vi "get_max_min.vi"(8 "error in":errorcluster, 11 "PI P123.01 & PiezoDrive TD250 & NI USB 7855R.lvclass":refnum<class "PI P123.01 & PiezoDrive TD250 & NI USB 7855R.lvclass">) -> (0 "error out":errorcluster, 1 "Piezo_minimum":i16, 2 "Piezo_maximum":i16, 3 "PI P123.01 & PiezoDrive TD250 & NI USB 7855R.lvclass 2":refnum<class "PI P123.01 & PiezoDrive TD250 & NI USB 7855R.lvclass">)   [LabVIEW 2020, in "PI P123.01 & PiezoDrive TD250 & NI USB 7855R.lvclass"]
uses:
  PI P123.01 & PiezoDrive TD250 & NI USB 7855R.lvclass
  PI P123.01 & PiezoDrive TD250 & NI USB 7855R.lvclass/PI P123.01 & PiezoDrive TD250 & NI USB 7855R.ctl
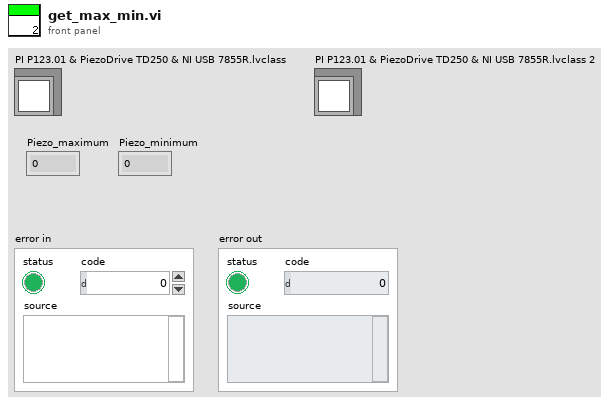
[diagram p1: front panel]
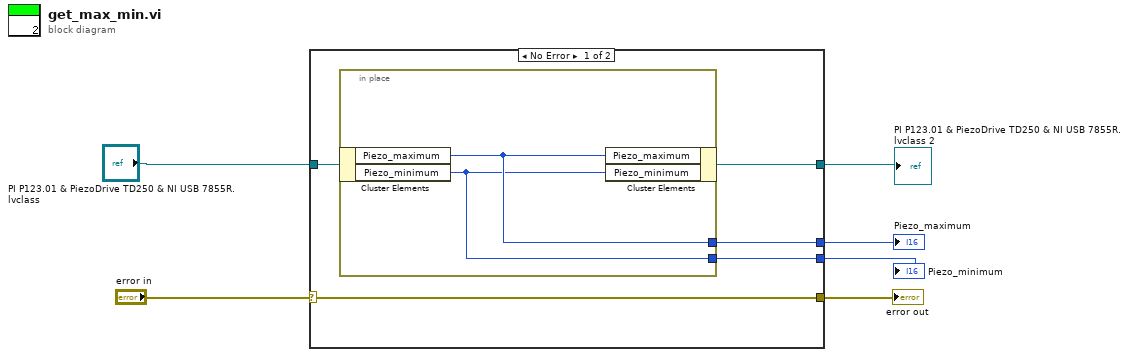
[diagram p0: block diagram]
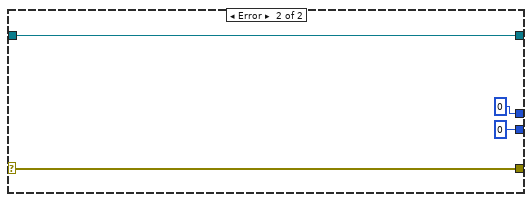
[diagram p2: hidden frame]
diagram:
  n1 = case shown="No Error" "error in" {
    selector: "error in" -> [w9 w16]
    tunnel: "PI P123.01 & PiezoDrive TD250 & NI USB 7855R.lvclass" -> [w11 w17]
    tunnel: [w10 w17] -> w5
    tunnel: [w9 w16] -> w3
    tunnel: [w8 i16 0 ("Piezo_maximum")] -> w2
    tunnel: [w7 i16 0 ("Piezo_minimum")] -> w1
    frame No Error {
      n2 = in-place {
        in-place-border: [w13] -> w8
        in-place-border: [w12] -> w7
        n3 = in-place-cluster #1(w11) -> ("Piezo_maximum"=w13:i16, "Piezo_minimum"=w12:i16)
        n4 = in-place-cluster #1("Piezo_maximum"=w13, "Piezo_minimum"=w12) -> (w10:refnum<class "PI P123.01 & PiezoDrive TD250 & NI USB 7855R.lvclass">)
      }
    }
    frame Error {
    }
  }
  "PI P123.01 & PiezoDrive TD250 & NI USB 7855R.lvclass 2" <- w5
  "error out" <- w3
  "Piezo_maximum" <- w2
  "Piezo_minimum" <- w1
